vi "oa_Interpolation with CIC and Compensation Filter.vi"(0 "x[n]":dbl[](array[numeric]) format="%.2f", 5 "CIC interpolation setting":T2, 7 "interpolation filters":T1[](array[typedef]) {"coefficients" format="%.2f"}, 11 "error in (no error)":errorcluster, 12 "state in":cluster{cluster{dbl[]}, cluster{dbl[]}[]}) -> (4 "x[n] out":dbl[](array[numeric]) format="%.2f", 14 "state out":cluster{cluster{dbl[]}, cluster{dbl[]}[]}, 15 "error out":errorcluster)   [LabVIEW 2017, in "SoundVib_Resampling.lvlib"]
uses:
  <vilib>/addons/Sound and Vibration/Order Analysis/Resample Order Tracking/SoundVib_Resampling.lvlib
  <vilib>/addons/_NISVFA/_Shared subVIs/Controls/OAT Decimation Filter.ctl
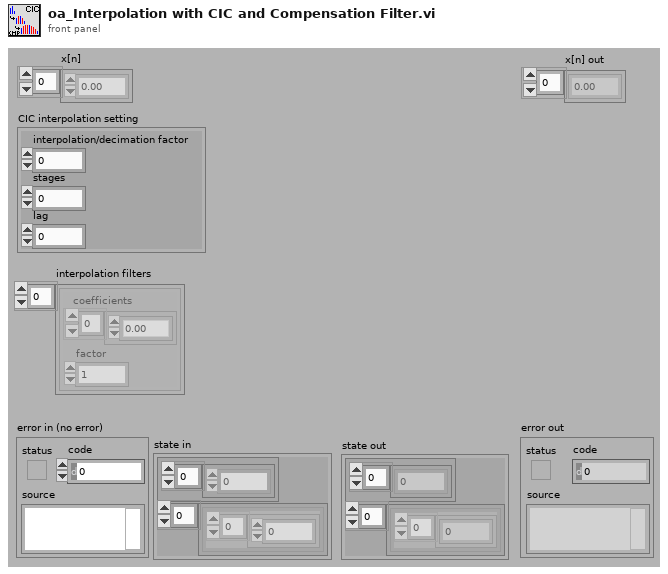
[diagram p1: front panel]
types:
  T1 = typedef "OAT Decimation Filter.ctl" = cluster{"coefficients":dbl[], "factor":i32}
  T2 = cluster{"interpolation/decimation factor":i32, "stages":i32, "lag":i32}
  T3 = cluster{"interpolation/decimation factor":i32, "stages":i32, "lag":i32}[]
  T4 = cluster{cluster{"final state":dbl[]}, "final state":cluster{"final state":dbl[]}[]}
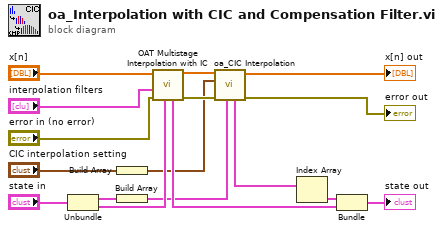
[diagram p0: block diagram]
diagram:
  n1 = Unbundle("state in") -> (w14:cluster{dbl[]}, w12:cluster{dbl[]}[])
  n2 = Build Array("CIC interpolation setting") -> (w7:T3)
  n3 = Build Array(w14) -> (w6:cluster{dbl[]}[])
  n4 = call <vilib>:"OAT Multistage Interpolation with IC.vi"("initial state"=w12, "error in (no error)"="error in (no error)", "filter"="interpolation filters", "X"="x[n]") -> ("error out"=w8:errorcluster, "Y"=w9:dbl[], "final state"=w11:cluster{"final state":dbl[]}[])  [unwired: 5 in]
  n5 = call <vilib>:"oa_CIC Interpolation.vi"("initial state"=w6, "error in (no error)"=w8, "CIC filter settings"=w7, "X"=w9) -> ("error out"=→"error out":errorcluster, "Y"=→"x[n] out":dbl[], "final state"=w5:cluster{"final state":dbl[]}[])  [unwired: 5 in]
  n6 = Index Array(array=w5) -> (element=w16:cluster{"final state":dbl[]})  [unwired: 1 in]
  n7 = Bundle(w16, "final state"=w11) -> (→"state out":T4)  [unwired: 1 in]
